vi "Begin.vi"(8 "error in":errorcluster) -> (0 "error out":errorcluster)   [LabVIEW 2016]
doc: "Called before other user functions, this VI is expected to open initial I/O refnums, load in file data, and do all program initialization. Notice that the <B>error out</B> terminal is simply used for data flow. Wiring it to other structures or subVIs ensures that this VI runs first."
uses:
  <vilib>/Rock Robotics/WPI/DriverStation/WPI_DriverStationRobotMode2.ctl
  <vilib>/Rock Robotics/SystemInterfaces/AI/FPGA_AIGyroChannel.ctl
  <vilib>/Rock Robotics/SystemInterfaces/DIO/FPGA_DIOChannel.ctl
  Sprocket/src/Refname/Sensors.ctl
  Sprocket/src/Refname/Actuators.ctl
  <vilib>/Rock Robotics/WPI/Solenoid/WPI_SolenoidChannel.ctl
  Sprocket/src/Refname/Joysticks.ctl
  <vilib>/Rock Robotics/WPI/Joystick/WPI_JoystickDeviceEnum.ctl
  Sprocket/src/Refname/Queues.ctl
  <vilib>/Rock Robotics/WPI/SafetyOutput/WPI_SafetyOutputConfigMenu.ctl
  <vilib>/Rock Robotics/WPI/ThirdParty/CanMotor/TalonSRX/WPI_CANTalonSRX_APIControlMode.ctl
  <vilib>/Rock Robotics/WPI/ThirdParty/CanMotor/TalonSRX/WPI_CANTalonSRX_APIFeedbackSelect.ctl
  Sprocket/src/Refname/Refname to String (Queue).vi
  Sprocket/src/Refname/Refname to String (Actuator).vi
  Sprocket/src/Refname/Refname to String (Sensor).vi
  Robot Global Data.vi
  <vilib>/Rock Robotics/WPI/Gyro/WPI_GyroAnalogOpen.vi
  <vilib>/Rock Robotics/WPI/Switch/WPI_SwitchOpenLimit.vi
  <vilib>/Rock Robotics/WPI/Solenoid/WPI_SolenoidOpenSingle.vi
  Sprocket/lib/Sprocket.lvlib
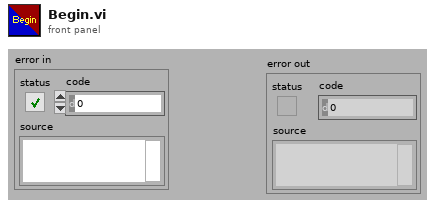
[diagram p1: front panel]
types:
  T1 = typedef "Sprocket.lvlib/Queues.ctl" = enum16{"Input", "Drive", "Collector", "Shifter", "Wedge"}
  T2 = typedef "Sprocket.lvlib/Joysticks.ctl" = enum16{"Joystick 0", "Joystick 1", "Joystick 2", "Joystick 3"}
  T3 = typedef "WPI_JoystickDeviceEnum.ctl" = enum16{"USB 0", "USB 1", "USB 2", "USB 3", "USB 4", "USB 5"}
  T4 = cluster{"Joystick Refname":T2, "JoystickDevice":T3}[]
  T5 = typedef "Sprocket.lvlib/Actuators.ctl" = enum16{"Drive Motor 1 (R)", "Drive Motor 2 (R)", "Drive Motor 3 (R)", "Drive Motor 4 (L)", "Drive Motor 5 (L)", "Drive Motor 6 (L)", "Collector Motor", "Collector Solenoid", "Compressor", "SonicShifter", "Gyro", "UltraSonic Front Left", "UltraSonic Back Left", "Wedge Motor", "Wedge LS"}
  T6 = cluster{"Actuator":T5, "CAN ID":u8, "Invert?":bool}[]
  T7 = typedef "WPI_SolenoidChannel.ctl" = enum8{"Solenoid 0", "Solenoid 1", "Solenoid 2", "Solenoid 3", "Solenoid 4", "Solenoid 5", "Solenoid 6", "Solenoid 7", "Invalid"}
  T8 = typedef "Sprocket.lvlib/Sensors.ctl" = enum16{"DIP 1", "DIP 2", "DIP 3", "DIP 4"}
  T9 = typedef "FPGA_DIOChannel.ctl" = enum8{"DIO 0", "DIO 1", "DIO 2", "DIO 3", "DIO 4", "DIO 5", "DIO 6", "DIO 7", "DIO 8", "DIO 9", "DIO MXP 0", "DIO MXP 1", "DIO MXP 2", "DIO MXP 3", "DIO MXP 4", "DIO MXP 5", "DIO MXP 6", "DIO MXP 7", "DIO MXP 8", "DIO MXP 9", "DIO MXP 10", "DIO MXP 11", "DIO MXP 12", "DIO MXP 13", "DIO MXP 14", "DIO MXP 15", "SPI Port CS1", "SPI Port CS2", "SPI Port CS3", "SPI Port MISO", "SPI Port MOSI", "Invalid"}
  T10 = typedef "FPGA_AIGyroChannel.ctl" = enum8{"AI 0", "AI 1", "Invalid"}
  T11 = typedef "WPI_DriverStationRobotMode2.ctl" = enum16{"Autonomous Disabled", "Autonomous Enabled", "Teleop Disabled", "Teleop Enabled", "Disconnected", "Finish", "Test Disabled", "Test Enabled", "Emergency Stopped"}
  T12 = typedef "WPI_CANTalonSRX_APIControlMode.ctl" = enum8{"Percent VBus", "Speed", "Position", "Slave", "Unchanged / Invalid", "Voltage Compensation", "Current", "Motion Profile", "Motion Magic"}
  T13 = typedef "WPI_SafetyOutputConfigMenu.ctl" = enum16{"Enable", "Disable"}
  T14 = typedef "WPI_MotorControlDeviceRef.ctl" = cluster{"DeviceStatus":errorcluster, "Type":T15, "PWM":cluster{"PWM Channel":T16, "DeadBand":T17}, "CAN":cluster{"Device Number":u8, "SetOutput VI Ref":variant, "GetOutput VI Ref":variant, "Enable VI Ref":variant, "Disable VI Ref":variant, "Data":variant}, "Invert":bool}
  T15 = typedef "WPI_MotorControlType.ctl" = enum16{"PWM", "CAN"}
  T16 = typedef "FPGA_DIOPWMChannel.ctl" = enum8{"PWM 0", "PWM 1", "PWM 2", "PWM 3", "PWM 4", "PWM 5", "PWM 6", "PWM 7", "PWM 8", "PWM 9", "PWM MXP 0", "PWM MXP 1", "PWM MXP 2", "PWM MXP 3", "PWM MXP 4", "PWM MXP 5", "PWM MXP 6", "PWM MXP 7", "PWM MXP 8", "PWM MXP 9", "Invalid"}
  T17 = typedef "WPI_PWMDeadband.ctl" = cluster{"Name":string, "maxPositivePwm":i32, "minPositivePwm":i32, "centerPwm":i32, "maxNegativePwm":i32, "minNegativePwm":i32, "angularRange":u16}
  T18 = typedef "WPI_SolenoidDevRef.ctl" = cluster{"DevStatus":errorcluster, "Pneumatics Control Module":u8, "Forward Solenoid Channel":T7, "Reverse Solenoid Channel":T7}
  T19 = typedef "WPI_SwitchDevRef.ctl" = cluster{"DevStatus":errorcluster, "DIO Channel":T9, "CntIndex":T20, "Normally Closed":bool}
  T20 = typedef "FPGA_CounterCtrSystemIndex.ctl" = enum8{"Ctr 0", "Ctr 1", "Ctr 2", "Ctr 3", "Ctr 4", "Ctr 5", "Ctr 6", "Ctr 7", "Invalid"}
  T21 = typedef "WPI_GyroDevRef.ctl" = cluster{"DevStatus":errorcluster, "Analog Channel":T22, "Offset":dbl, "Gain (VoltsPerDegree/Second)":dbl, "Gyro Type":enum16{"Analog", "XRS450"}, "Handle":i32, "SPI Bus":T23, "Device Found":bool, "Sample Rate":dbl, "Calibrate On Open":bool}
  T22 = typedef "FPGA_AIChannel.ctl" = enum8{"AI 0", "AI 1", "AI 2", "AI 3", "AI MXP 0", "AI MXP 1", "AI MXP 2", "AI MXP 3", "Invalid"}
  T23 = typedef "spi_bus.ctl" = enum16{"SPI On-Board, CS0", "SPI On-Board, CS1", "SPI On-Board, CS2", "SPI On-Board, CS3", "SPI MXP", "Invalid"}
  T24 = typedef "WPI_JoystickDevRef.ctl" = cluster{"Device":T3}
  T25 = typedef "WPI_CANTalonSRX_APIFeedbackSelect.ctl" = enum16{"Digital Quadrature Encoder", "Analog Potentiometer", "Analog Encoder", "Count on Quad-A (Rising-Edge)", "Count on Quad-A (Falling-Edge)", "CTR Magnetic Enc (Absolute)", "CTR Magnetic Enc (Relative)", "Pulse Width"}
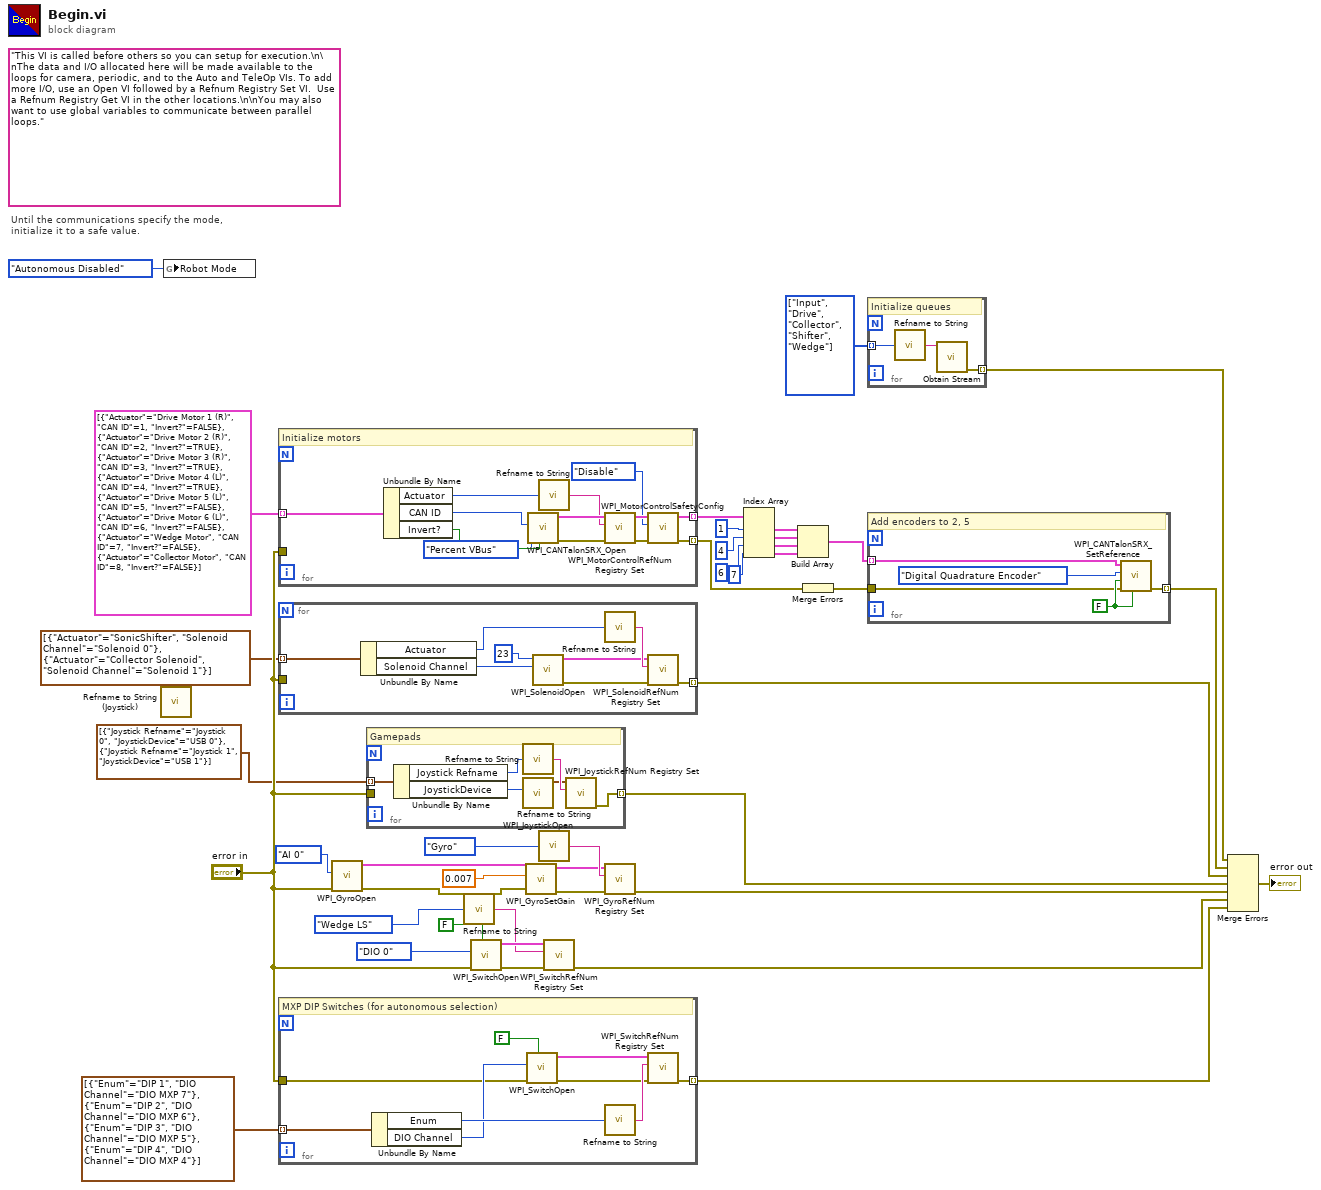
[diagram p0: block diagram]
diagram:
  w5 = T1[] [enum."Input", enum."Drive", enum."Collector", enum."Shifter", enum."Wedge"] items=["Input", "Drive", "Collector", "Shifter", "Wedge"]
  (unwired) "This VI is called before others so you can setup for execution.\n\nThe data and I/O allocated here will be made available to the loops for camera, periodic, and to the Auto and TeleOp VIs. To add more I/O, use an Open VI followed by a Refnum Registry Set VI.  Use a Refnum Registry Get VI in the other locations.\n\nYou may also want to use global variables to communicate between parallel loops."
  # "Until the communications specify the mode,\ninitialize it to a safe value."
  n1 = call "Refname to String (Joystick).vi"() -> ()  [unwired: 1 in, 1 out]
  n2 = global write "Robot Global Data.vi" "Robot Mode"(WPI_DriverStationRobotMode2."Autonomous Disabled" ("Robot Mode")) -> ()
  n3 = for {
    tunnel: [w54] -> w19 mode=indexing
    tunnel: T6 [{"Actuator"=enum."Drive Motor 1 (R)", "CAN ID"=1, "Invert?"=FALSE}, {"Actuator"=enum."Drive Motor 2 (R)", "CAN ID"=2, "Invert?"=TRUE}, {"Actuator"=enum."Drive Motor 3 (R)", "CAN ID"=3, "Invert?"=TRUE}, {"Actuator"=enum."Drive Motor 4 (L)", "CAN ID"=4, "Invert?"=TRUE}, {"Actuator"=enum."Drive Motor 5 (L)", "CAN ID"=5, "Invert?"=FALSE}, {"Actuator"=enum."Drive Motor 6 (L)", "CAN ID"=6, "Invert?"=FALSE}, {"Actuator"=enum."Wedge Motor", "CAN ID"=7, "Invert?"=FALSE}, {"Actuator"=enum."Collector Motor", "CAN ID"=8, "Invert?"=FALSE}] -> [w46] mode=indexing
    tunnel: [w53] -> w17 mode=indexing
    tunnel: "error in" -> [_]
    # "Initialize motors"
    n4 = Unbundle By Name(w46) -> ("Actuator"=w48:T5, "CAN ID"=w43:u8, "Invert?"=w47:bool)
    n5 = call <vilib>:"WPI_CANTalonSRX_Open.vi"("Invert"=w47, "Device Number"=w43, "Control Mode"=WPI_CANTalonSRX_APIControlMode."Percent VBus") -> ("error out"=w50:errorcluster, "CAN Talon SRX Ref"=w49:T14)  [unwired: 7 in]
    n6 = call-poly "Refname to String.vi"("Actuator Refname"=w48) -> ("Refnum Name"=w45:string)
    n7 = call <vilib>:"WPI_MotorControlRefNum Registry Set.vi"("error in (no error)"=w50, "refnum name"=w45, "MotorControlDevRef"=w49) -> ("error out"=w52:errorcluster, "MotorControlDevRef"=w51:T14)  [unwired: 7 in]
    n8 = call <vilib>:"WPI_MotorControlSafetyConfig.vi"("error in (no error)"=w52, "mode"=WPI_SafetyOutputConfigMenu."Disable", "MotorControlDevRef"=w51) -> ("error out"=w54:errorcluster, "MotorControlDevRef"=w53:T14)  [unwired: 7 in]
  }
  n9 = for {
    tunnel: cluster{"Actuator":T5, "Solenoid Channel":T7}[] [{"Actuator"=enum."SonicShifter", "Solenoid Channel"=enum."Solenoid 0"}, {"Actuator"=enum."Collector Solenoid", "Solenoid Channel"=enum."Solenoid 1"}] -> [w62] mode=indexing
    tunnel: [w58] -> w23 mode=indexing
    tunnel: "error in" -> [_]
    n10 = Unbundle By Name(w62) -> ("Actuator"=w61:T5, "Solenoid Channel"=w60:T7)
    n11 = call-poly <vilib>:"WPI_SolenoidOpen.vi"("Solenoid Channel"=w60, "Pneumatics Control Module (0)"=u8 23) -> ("error out"=w57:errorcluster, "SolenoidDevRef"=w56:T18)  [unwired: 8 in]
    n12 = call-poly "Refname to String.vi"("Actuator Refname"=w61) -> ("Refnum Name"=w59:string)
    n13 = call <vilib>:"WPI_SolenoidRefNum Registry Set.vi"("error in (no error)"=w57, "refnum name"=w59, "SolenoidDevRef"=w56) -> ("error out"=w58:errorcluster)  [unwired: 7 in, 1 out]
  }
  n14 = for {
    tunnel: cluster{"Enum":T8, "DIO Channel":T9}[] [{"Enum"=enum."DIP 1", "DIO Channel"=enum."DIO MXP 7"}, {"Enum"=enum."DIP 2", "DIO Channel"=enum."DIO MXP 6"}, {"Enum"=enum."DIP 3", "DIO Channel"=enum."DIO MXP 5"}, {"Enum"=enum."DIP 4", "DIO Channel"=enum."DIO MXP 4"}] -> [w71] mode=indexing
    tunnel: "error in" -> [w65]
    tunnel: [w63] -> w9 mode=indexing
    # "MXP DIP Switches (for autonomous selection)"
    n15 = Unbundle By Name(w71) -> ("Enum"=w70:T8, "DIO Channel"=w69:T9)
    n16 = call-poly <vilib>:"WPI_SwitchOpen.vi"("Normally Closed"=FALSE, "error in (no error)"=w65, "DIO Channel"=w69) -> ("error out"=w64:errorcluster, "SwitchDevRef"=w68:T19)  [unwired: 7 in]
    n17 = call-poly "Refname to String.vi"("Sensor Refname"=w70) -> ("Refnum Name"=w67:string)
    n18 = call <vilib>:"WPI_SwitchRefNum Registry Set.vi"("error in (no error)"=w64, "refnum name"=w67, "SwitchDevRef"=w68) -> ("error out"=w63:errorcluster)  [unwired: 7 in, 1 out]
  }
  n19 = call-poly <vilib>:"WPI_GyroOpen.vi"("error in (no error)"="error in", "Analog Channel"=FPGA_AIGyroChannel."AI 0") -> ("error out"=w31:errorcluster, "GyroDevRef"=w32:T21)  [unwired: 7 in, 1 out]
  n20 = for {
    tunnel: T4 [{"Joystick Refname"=enum."Joystick 0", "JoystickDevice"=enum."USB 0"}, {"Joystick Refname"=enum."Joystick 1", "JoystickDevice"=enum."USB 1"}] -> [w77] mode=indexing
    tunnel: [w74] -> w7 mode=indexing
    tunnel: "error in" -> [_]
    # "Gamepads"
    n21 = Unbundle By Name(w77) -> ("Joystick Refname"=w72:T2, "JoystickDevice"=w76:T3)
    n22 = call-poly "Refname to String.vi"("Joystick Refname"=w72) -> ("Refnum Name"=w75:string)
    n23 = call <vilib>:"WPI_JoystickOpen.vi"("JoystickDevice"=w76) -> ("JoystickDevRef"=w73:T24)  [unwired: 10 in]
    n24 = call <vilib>:"WPI_JoystickRefNum Registry Set.vi"("refnum name"=w75, "JoystickDevRef"=w73) -> ("error out"=w74:errorcluster)  [unwired: 8 in, 1 out]
  }
  n25 = call-poly "Refname to String.vi"("Actuator Refname"=Actuators."Wedge LS") -> ("Refnum Name"=w33:string)
  n26 = call-poly <vilib>:"WPI_SwitchOpen.vi"("Normally Closed"=FALSE, "error in (no error)"="error in", "DIO Channel"=FPGA_DIOChannel."DIO 0") -> ("error out"=w34:errorcluster, "SwitchDevRef"=w35:T19)  [unwired: 7 in]
  n27 = call <vilib>:"WPI_GyroSetGain.vi"("error in (no error)"=w31, "Gain (VoltsPerDegree/Second)"=0.007, "GyroDevRef"=w32) -> ("error out"=w30:errorcluster, "GyroDevRef"=w29:T21)  [unwired: 7 in]
  n28 = call-poly "Refname to String.vi"("Actuator Refname"=Actuators."Gyro") -> ("Refnum Name"=w39:string)
  n29 = call <vilib>:"WPI_SwitchRefNum Registry Set.vi"("error in (no error)"=w34, "refnum name"=w33, "SwitchDevRef"=w35) -> ("error out"=w3:errorcluster)  [unwired: 7 in, 1 out]
  n30 = call <vilib>:"WPI_GyroRefNum Registry Set.vi"("error in (no error)"=w30, "refnum name"=w39, "GyroDevRef"=w29) -> ("error out"=w4:errorcluster)  [unwired: 7 in, 1 out]
  n31 = Index Array(array=w17, index #1=1 ("index"), index #2=4 ("index"), index #3=6 ("index"), index #4=7 ("index")) -> (element #1=w16:T14, element #2=w15:T14, element #3=w14:T14, element #4=w1:T14)
  n32 = Build Array(w16, w15, w14, w1) -> (w10:T14[])
  n33 = Merge Errors(w19) -> (w20:errorcluster)
  n34 = for {
    tunnel: w5 -> [w78] mode=indexing
    tunnel: [w80] -> w6 mode=indexing
    # "Initialize queues"
    n35 = call-poly "Refname to String.vi"("Queue Refname"=w78) -> ("Refnum Name"=w79:string)
    n36 = call "Obtain Stream.vi"("Name"=w79) -> ("error out"=w80:errorcluster)  [unwired: 9 in, 1 out]
  }
  n37 = for {
    tunnel: w10 -> [w85] mode=indexing
    tunnel: [w82] -> w21 mode=indexing
    tunnel: w20 -> [w81]
    w83 = FALSE
    # "Add encoders to 2, 5"
    n38 = call <vilib>:"WPI_CANTalonSRX_SetReference.vi"("Reverse Closed-Loop Output"=w83, "error in (no error)"=w81, "Reverse Feedback Sensor"=w83, "Feedback Reference"=WPI_CANTalonSRX_APIFeedbackSelect."Digital Quadrature Encoder", "CAN Talon SRX Ref"=w85) -> ("error out"=w82:errorcluster)  [unwired: 5 in, 1 out]
  }
  n39 = Merge Errors(w6, w21, w23, w7, w4, w3, w9) -> (→"error out":errorcluster)
